vi "Tokenize  JSON String.vi"(10 "JSON String":string) -> (2 "Value Tokens":cluster{"Token Type":T1, "Token Value":string}[](array[cluster]))   [LabVIEW 2015, in "LVJSON.lvlib" / "JSON Datatype.lvclass"]
uses:
  JSON Data Classes/JSON Datatype/JSON Datatype.lvclass
  Token Types.ctl
  LVJSON.lvlib
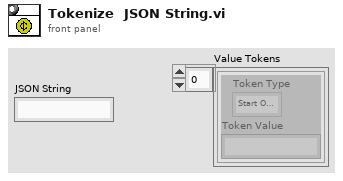
[diagram p1: front panel]
types:
  T1 = typedef "LVJSON.lvlib/Token Types.ctl" = enum32{"Start Object", "End Object", "Start Array", "End Array", "Quotation", "Numeric", "true", "false", "null", "Escape", "Undefined"}
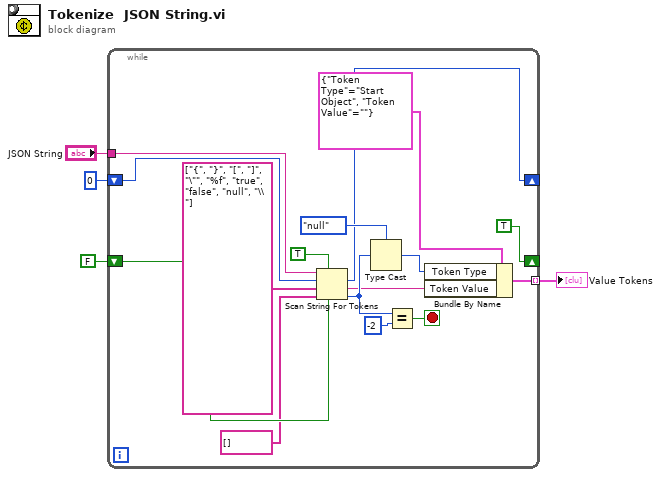
[diagram p0: block diagram]
diagram:
  n1 = while {
    tunnel: "JSON String" -> [w20]
    shift-right: [w10] -> _
    shift-left: 0 ("offset past token") -> [w11]
    shift-right: [TRUE] -> _
    shift-left: FALSE -> [w9]
    tunnel: [w7] -> w1 mode=indexing
    stop <- w16 stop-if-true
    n2 = Scan String For Tokens(4:w9, 5:TRUE ("allow empty tokens? (F)"), 6:string[] [] ("delimiters (\\s,\\t,\\r,\\n)"), 7:string[] ["{", "}", "[", "]", "\"", "%f", "true", "false", "null", "\\"] ("operators (none)"), 8:w11, 9:w20) -> (0:w13:i32, 1:w12:string, 2:w10:i32)  [unwired: 1 out]
    n3 = Type Cast(type=Token_Types."null" ("Enum"), x=w13) -> (*(type *) &x=w6:T1)
    n4 = Equal?(x=w13, y=-2) -> (x = y?=w16:bool)
    n5 = Bundle By Name(cluster=cluster{"Token Type":T1, "Token Value":string} {"Token Type"=enum."Start Object", "Token Value"=""} ("input cluster"), "Token Type"=w6, "Token Value"=w12) -> (w7:cluster{"Token Type":T1, "Token Value":string})
  }
  "Value Tokens" <- w1
